vi "data sorting results simple.vi"(8 "error in":errorcluster, 11 "cycle results cluster IN":T1) -> (0 "error out":errorcluster, 3 "cycle results cluster out":T1)   [LabVIEW 2016]
doc: "Takes a sample type and sorts by sequence"
uses:
  controls/cycle results control.ctl
  <vilib>/Analysis/baseanly.llb/Mean (DBL).vi
  <vilib>/Analysis/NI_AALBase.lvlib
panel:
  out "Array 4":string[](array[string])
  out "Array 2":dbl[][][](array[numeric])
  out "subarray":string[](array[string])
  out "Array":dbl[][](array[numeric])
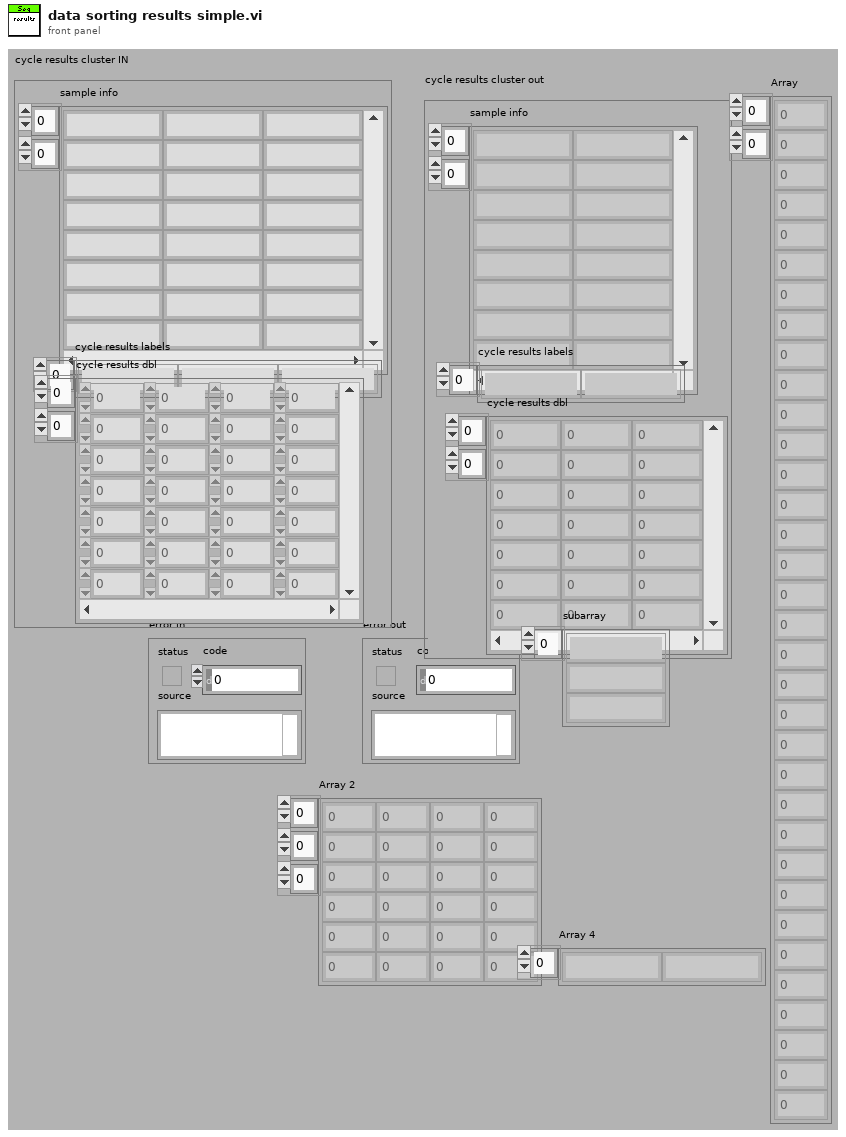
[diagram p1: front panel]
types:
  T1 = typedef "cycle results control.ctl" = cluster{"sample info":string[][], "cycle results labels":string[], "cycle results dbl":dbl[][]}
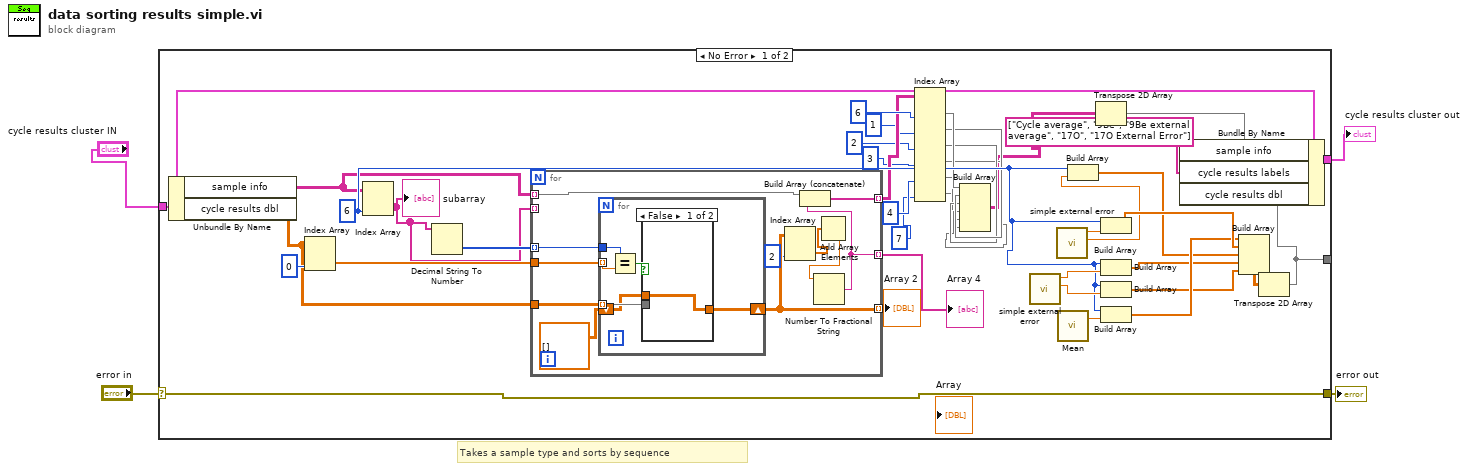
[diagram p0: block diagram]
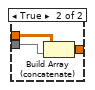
[diagram p2: hidden frame]
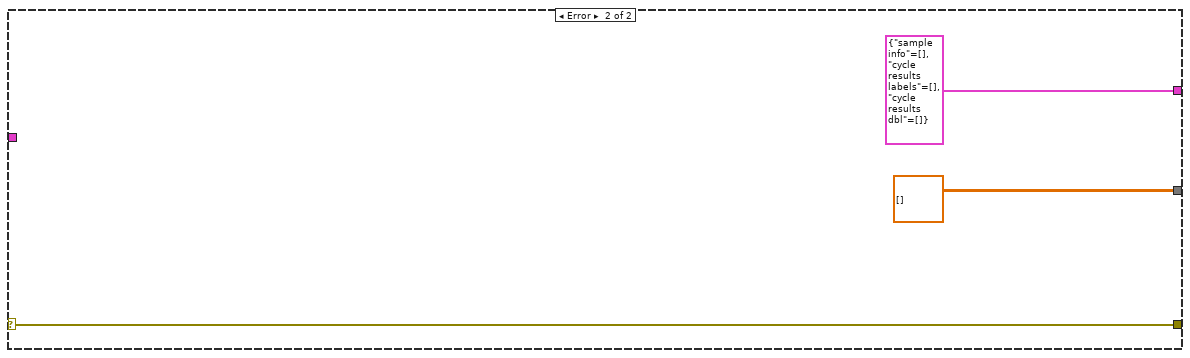
[diagram p3: hidden frame]
diagram:
  # "Takes a sample type and sorts by sequence"
  n1 = case shown="No Error" "error in" {
    selector: "error in" -> [w41 w67]
    tunnel: "cycle results cluster IN" -> [w40 _]
    tunnel: [w36 dbl[][] []] -> _
    tunnel: [w38 T1 {"sample info"=[], "cycle results labels"=[], "cycle results dbl"=[]} ("cycle results cluster IN")] -> w2
    tunnel: [w41 w67] -> w3
    frame No Error {
      w28 = 6 ("disabled index (col)")
      n2 = Unbundle By Name(w40) -> ("sample info"=w20:string[][], "cycle results dbl"=w24:dbl[][])
      n3 = Index Array(array=w24, index (col)=0 ("disabled index (col)")) -> (element=w26:dbl[])  [unwired: 1 in]
      n4 = Index Array(array=w20, index (col)=w28) -> (element=w22:string[])  [unwired: 1 in]
      "subarray" <- w22
      n5 = Decimal String To Number(string=w22) -> (number=w25:i32[])  [unwired: 2 in, 1 out]
      n6 = for {
        tunnel: w26 -> [w55]
        tunnel: w25 -> [w54] mode=indexing
        tunnel: w24 -> [w53]
        tunnel: [w51] -> w23 mode=indexing
        tunnel: w22 -> [_] mode=indexing
        tunnel: [w47] -> w21 mode=indexing
        tunnel: [w46] -> w10 mode=indexing
        tunnel: w20 -> [w45] mode=indexing
        n7 = for {
          tunnel: w55 -> [w61] mode=indexing
          tunnel: w54 -> [w60]
          tunnel: w53 -> [w58] mode=indexing
          shift-right: [w57] -> w51
          shift-left: dbl[][] [] -> [w56]
          n8 = Equal?(x=w60, y=w61) -> (x = y?=w59:bool)
          n9 = case shown="False" w59 {
            tunnel: w58 -> [_ w65]
            tunnel: [w62 w64] -> w57
            tunnel: w56 -> [w62 w63]
            frame False {
            }
            frame True {
              n10 = Build Array (concatenate)(w63, w65) -> (w64:dbl[][])
            }
          }
        }
        n11 = Index Array(array=w51, index (col)=2 ("disabled index (col)")) -> (element=w49:dbl[])  [unwired: 1 in]
        n12 = Add Array Elements(numeric array=w49) -> (sum=w48:dbl)
        n13 = Number To Fractional String(number=w48) -> (F-format string=w47:string)  [unwired: 3 in]
        n14 = Build Array (concatenate)(w45, w47) -> (w46:string[])
      }
      "Array 2" <- w23
      "Array 4" <- w21
      n15 = Index Array(array=w10, index (col) #1=6 ("disabled index (col)"), index (col) #2=1 ("disabled index (row)"), index (col) #3=2 ("index (row)"), index (col) #4=3 ("disabled index (col)"), index (col) #5=4 ("index (col)"), index (col) #6=7 ("index (col)")) -> (element #1=w18:string[], element #2=w17:string[], element #3=w16:string[], element #4=w15:string[], element #5=w14:string[], element #6=w13:string[])  [unwired: 6 in]
      n16 = Build Array(w18, w17, w16, w15, w14, w13) -> (w12:string[][])
      n17 = call "simple external error.vi"() -> ("External error"=w32:dbl, "Sequence result"=w33:dbl)  [unwired: 8 in, 2 out]
      n18 = call "simple external error.vi"() -> ("External error"=w34:dbl, "Sequence result"=w35:dbl)  [unwired: 8 in, 2 out]
      n19 = call-poly <vilib>:"Mean.vi"() -> ("mean"=w44:dbl)  [unwired: 1 in, 1 out]
      n20 = Build Array(w28, w34) -> (w31:dbl[])
      n21 = Transpose 2D Array(2D array=w12) -> (transposed array=w11:string[][])
      n22 = Build Array(w28, w35) -> (w43:dbl[])
      n23 = Build Array(w28, w33) -> (w30:dbl[])
      n24 = Build Array(w28, w32) -> (w29:dbl[])
      n25 = Build Array(w28, w44) -> (w42:dbl[])
      n26 = Build Array(w42, w43, w31, w30, w29) -> (w37:dbl[][])
      n27 = Transpose 2D Array(2D array=w37) -> (transposed array=w36:dbl[][])
      n28 = Bundle By Name(cluster=w40, "sample info"=w11, "cycle results labels"=string[] ["Cycle average", "9Be", "9Be external average", "17O", "17O External Error"], "cycle results dbl"=w36) -> (w38:T1)
    }
    frame Error {
    }
  }
  "error out" <- w3
  "cycle results cluster out" <- w2
